vi "Configure Combined Measurement.vi"(8 "error in (no error)":errorcluster, 10 "channels":u16[](array[ring]) items=["no gauge", "channel 1", "channel 2", "channel 3"], 11 "VGC in":refnum<class "PL Inficon VGC.lvclass">) -> (0 "error out":errorcluster, 1 "measured value":dbl, 2 "channels":u16[](array[ring]) items=["no gauge", "channel 1", "channel 2", "channel 3"], 3 "VGC out":refnum<class "PL Inficon VGC.lvclass">)   [LabVIEW 2015, in "PL Inficon VGC.lvclass"]
doc: "Configures combined pressure range measurement."
uses:
  PL Inficon VGC.lvclass
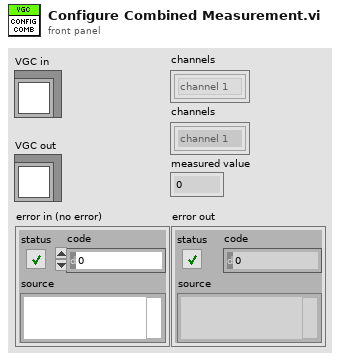
[diagram p1: front panel]
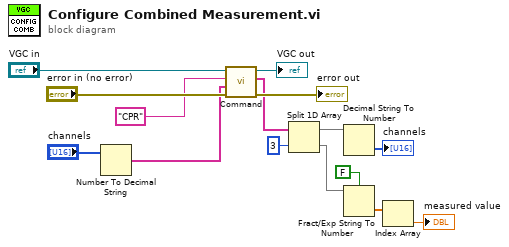
[diagram p0: block diagram]
diagram:
  n1 = Number To Decimal String(number="channels") -> (decimal integer string=w9:string[])  [unwired: 1 in]
  n2 = call "Command.vi"("error in (no error)"="error in (no error)", "parameters"=w9, "command"="CPR", "VGC in"="VGC in") -> ("error out"=→"error out":errorcluster, "response data"=w7:string[], "VGC out"=→"VGC out":refnum<class "PL Inficon VGC.lvclass">)  [unwired: 5 in]
  n3 = Split 1D Array(array=w7, index=3) -> (first subarray=w5:string[], second subarray=w4:string[])
  n4 = Decimal String To Number(string=w5) -> (number=→"channels":i32[])  [unwired: 2 in, 1 out]
  n5 = Fract/Exp String To Number(use system decimal point (T)=FALSE, string=w4) -> (number=w2:dbl[])  [unwired: 2 in, 1 out]
  n6 = Index Array(array=w2) -> (element=→"measured value":dbl)  [unwired: 1 in]
